vi "Thermometer_v2.vi"() -> ()   [LabVIEW 2023]
panel:
  in  "stop":bool
  in  "Skala temperatury":bool
  out "Temperatura [C]":dbl(slide) scale=0.0..100.0
  out "Temperatura [K":dbl(slide) scale=0.0..100.0
  # "Deg C"
  # "Deg K"
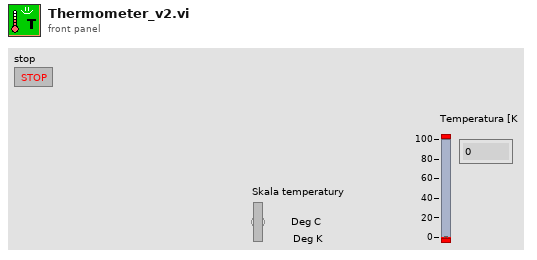
[diagram p1: front panel]
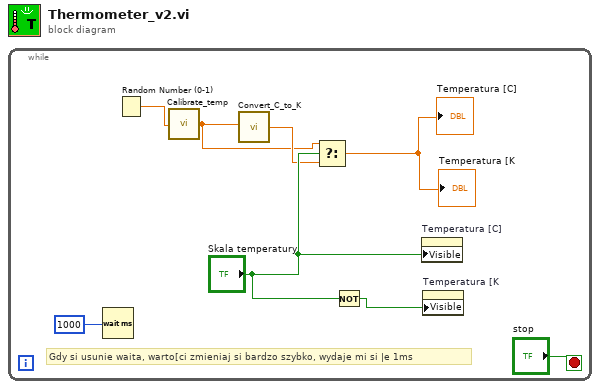
[diagram p0: block diagram]
diagram:
  n1 = while {
    stop <- "stop" stop-if-true
    # "Gdy si usunie waita, warto[ci zmieniaj si bardzo szybko, wydaje mi si |e 1ms"
    n2 = Wait (ms)(milliseconds to wait=1000) -> ()  [unwired: 1 out]
    n3 = Random Number (0-1)() -> (number: 0 to 1=w4:dbl)
    n4 = call "Calibrate_temp.vi"("Input"=w4) -> ("Output"=w2:dbl)
    n5 = call "Convert_C_to_K.vi"("deg C"=w2) -> ("deg K"=w3:dbl)
    n6 = Select(t=w2, s="Skala temperatury", f=w3) -> (s? t:f=→"Temperatura [K" →"Temperatura [C]":dbl)
    n7 = Not(x="Skala temperatury") -> (.not. x?=w7:bool)
    n8 = property on="Temperatura [C]" class="Slide (strict)"("Visible"="Skala temperatury") -> ()  [unwired: 2 in, 2 out]
    n9 = property on="Temperatura [K" class="Slide (strict)"("Visible"=w7) -> ()  [unwired: 2 in, 2 out]
  }
